vi "Read Config File.vi"(8 "error in (no error)":errorcluster, 11 "Config_Read_SPI.lvclass":refnum<class "Config_Read_SPI.lvclass">) -> (0 "error out":errorcluster, 3 "Config_Read_SPI.lvclass out":refnum<class "Config_Read_SPI.lvclass">)   [LabVIEW 2018, in "Config_Read_SPI.lvclass"]
uses:
  Config_Read_SPI.lvclass
  Config_Read_SPI.lvclass/Config_Read_SPI.ctl
  <vilib>/Utility/file.llb/Read Delimited Spreadsheet (string).vi
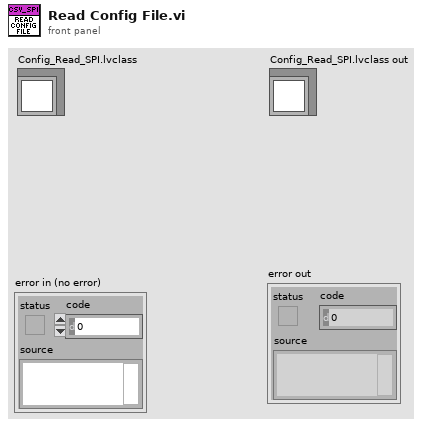
[diagram p1: front panel]
types:
  T1 = typedef "Config_Read_SPI.lvclass/SPI_FRM_Config.ctl" = cluster{"Pattern Name":string, "Data":u16, "Addr":u16, "R/W?":T2, "Opcode":string[], "SPI_Mode":T3}
  T2 = typedef "Config_Read_BML.lvclass/RW_Option.ctl" = enum16{"Read", "Write", "R/W"}
  T3 = typedef "Config_Read_SPI.lvclass/SPI_Mode.ctl" = enum16{"SPI_3W", "SPI_4W"}
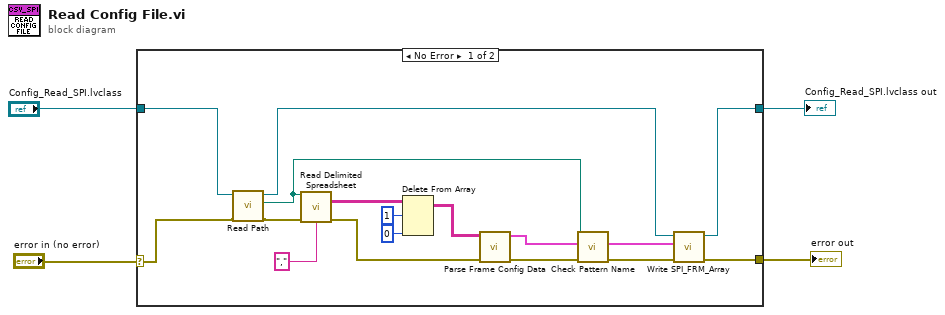
[diagram p0: block diagram]
diagram:
  n1 = case shown="No Error" "error in (no error)" {
    selector: "error in (no error)" -> [w16 w23]
    tunnel: [w8 w23] -> w3
    tunnel: [w5 w22] -> w1
    tunnel: "Config_Read_SPI.lvclass" -> [w17 w22]
    frame No Error {
      n2 = call "Read Path.vi"("error in (no error)"=w16, "Config_Read_SPI in"=w17) -> ("error out"=w15:errorcluster, "Path"=w11:path, "Config_Read_SPI out"=w7:refnum<class "Config_Read_SPI.lvclass">)  [unwired: 7 in]
      n3 = call-poly <vilib>:"Read Delimited Spreadsheet.vi"("file path (dialog if empty)"=w11, "error in (no error)"=w15, "delimiter (\\t)"="," ("delimiter (\\t)")) -> ("all rows"=w20:string[][], "error out"=w13:errorcluster)  [unwired: 7 in, 4 out]
      n4 = Delete From Array(array=w20, length=1, index (row)=0) -> (array with subset deleted=w14:string[][])  [unwired: 1 in, 1 out]
      n5 = call "Parse Frame Config Data.vi"("error in (no error)"=w13, "all rows"=w14) -> ("error out"=w12:errorcluster, "SPI FRM Config out"=w10:T1[])  [unwired: 8 in]
      n6 = call "Check Pattern Name.vi"("error in (no error)"=w12, "SPI FRM Config in"=w10, "Path"=w11) -> ("error out"=w9:errorcluster, "SPI FRM Config out"=w6:T1[])  [unwired: 7 in]
      n7 = call "Write SPI_FRM_Array.vi"("error in (no error)"=w9, "SPI_FRM_Array"=w6, "Config_Read_SPI in"=w7) -> ("error out"=w8:errorcluster, "Config_Read_SPI out"=w5:refnum<class "Config_Read_SPI.lvclass">)  [unwired: 7 in]
    }
    frame Error {
    }
  }
  "error out" <- w3
  "Config_Read_SPI.lvclass out" <- w1
